vi "nao_sonar.vi"(3 "error in":errorcluster, 4 "node":string, 5 "Side":enum16{"Left", "Right"}(ring)) -> (0 "error out":errorcluster, 2 "Range Data":T1)   [LabVIEW 2016]
doc: "Reads in the NAO's sonar"
uses:
  ROS/Code/Console/Servers/ServerSubs/TopicDef.ctl
  ROS/Code/SubVIs/_ROSDirection.ctl
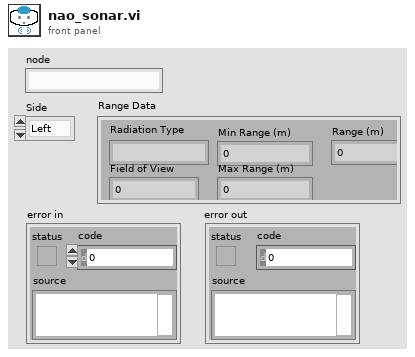
[diagram p1: front panel]
types:
  T1 = cluster{"Radiation Type":string, "Field of View":sgl, "Min Range (m)":sgl, "Max Range (m)":sgl, "Range (m)":sgl}
  T2 = typedef "TopicDef.ctl" = cluster{"Topic":string, "Type":string, "Action":T3, "Update (ms)":u16, "queue size":u16}
  T3 = typedef "_ROSDirection.ctl" = enum16{"Node", "Publisher", "Subscriber", "ServiceClient", "ServiceProvider"}
  T4 = typedef "_ROSControl.ctl" = cluster{"topic port":u16, "Node":string, "topic":string, "type":string, "node port":u16, "error ":errorcluster, "Direction":T3, "Update (ms)":u16, "FIFO size":u16}
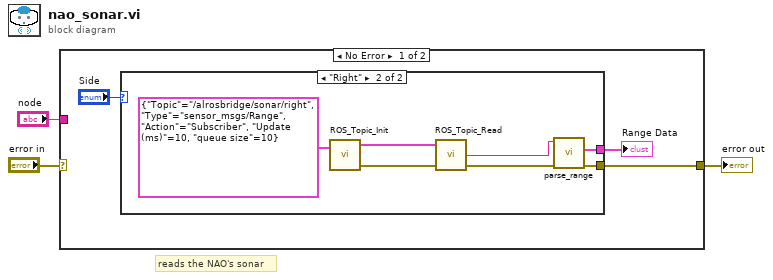
[diagram p0: block diagram]
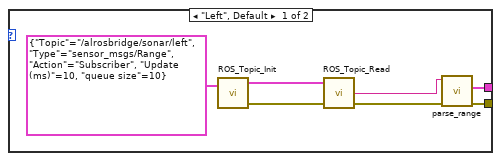
[diagram p2: hidden frame]
diagram:
  # "reads the NAO's sonar"
  n1 = case shown="No Error" "error in" {
    selector: "error in" -> [_ w21]
    tunnel: [w4 w21] -> w3
    tunnel: "node" -> [_ _]
    frame No Error {
      n2 = case shown="\"Right\"" "Side" {
        tunnel: [w8 w15] -> w5
        tunnel: [w7 w14] -> w4
        frame "Left", Default {
          n3 = call "ROS_Topic_Init.vi"("Definitions"=T2 {"Topic"="/alrosbridge/sonar/left", "Type"="sensor_msgs/Range", "Action"=enum."Subscriber", "Update (ms)"=10, "queue size"=10}) -> ("ROS out"=w13:T4, "error out"=w11:errorcluster)  [unwired: 2 in]
          n4 = call "ROS_Topic_Read.vi"("error in (no error)"=w11, "ROS in"=w13) -> ("error out"=w9:errorcluster, "Reply"=w10:string)  [unwired: 1 in, 1 out]
          n5 = call "parse_range.vi"("error in"=w9, "msg in"=w10) -> ("error out"=w7:errorcluster, "Range Data"=w8:T1)  [unwired: 2 in, 2 out]
        }
        frame "Right" {
          n6 = call "ROS_Topic_Init.vi"("Definitions"=T2 {"Topic"="/alrosbridge/sonar/right", "Type"="sensor_msgs/Range", "Action"=enum."Subscriber", "Update (ms)"=10, "queue size"=10}) -> ("ROS out"=w20:T4, "error out"=w18:errorcluster)  [unwired: 2 in]
          n7 = call "ROS_Topic_Read.vi"("error in (no error)"=w18, "ROS in"=w20) -> ("error out"=w16:errorcluster, "Reply"=w17:string)  [unwired: 1 in, 1 out]
          n8 = call "parse_range.vi"("error in"=w16, "msg in"=w17) -> ("error out"=w14:errorcluster, "Range Data"=w15:T1)  [unwired: 2 in, 2 out]
        }
      }
      "Range Data" <- w5
    }
    frame Error {
    }
  }
  "error out" <- w3
